vi "SetClosedChannels.vi"(7 "Slot":T1, 8 "Error In":errorcluster, 10 "Channels":bool[](array[boolean]), 11 "Keithley 7001 In":refnum<visa-resource-name>) -> (0 "Error Out":errorcluster, 3 "Keithley 7001 Out":refnum<visa-resource-name>)   [LabVIEW 2012, in "Keithley-7001.lvlib"]
uses:
  Keithley-7001.lvlib
  Controls/Slot.ctl
panel:
  # "33"
  # "34"
  # "35"
  # "1"
  # "2"
  # "3"
  # "4"
  # "5"
  # "6"
  # "7"
  # "8"
  # "9"
  # "10"
  # "11"
  # "12"
  # "13"
  # "14"
  # "15"
  # "16"
  # "17"
  # "18"
  # "19"
  # "20"
  # "21"
  # "22"
  # "23"
  # "24"
  # "25"
  # "26"
  # "27"
  # "28"
  # "29"
  # "30"
  # "31"
  # "32"
  # "36"
  # "37"
  # "38"
  # "39"
  # "40"
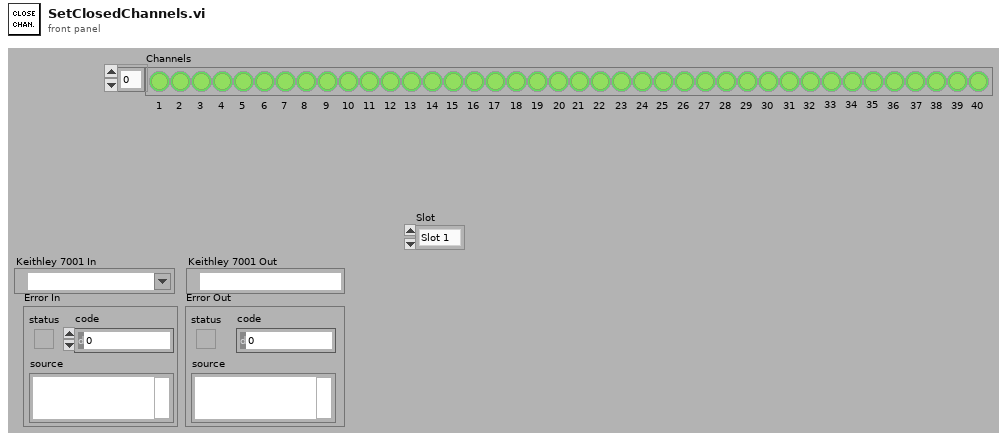
[diagram p1: front panel]
types:
  T1 = typedef "Keithley-7001.lvlib/Slot.ctl" = enum16{"Slot 1", "Slot 2"}
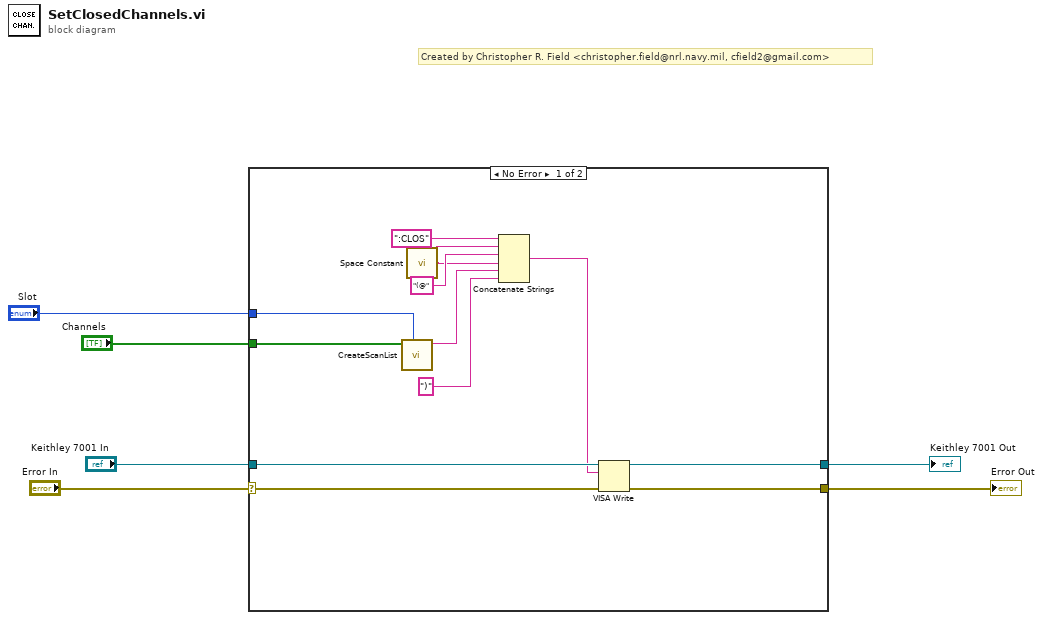
[diagram p0: block diagram]
diagram:
  # "Created by Christopher R. Field <christopher.field@nrl.navy.mil, cfield2@gmail.com>"
  n1 = case shown="No Error" "Error In" {
    selector: "Error In" -> [w8 w19]
    tunnel: "Keithley 7001 In" -> [w18 w20]
    tunnel: [w17 w20] -> w5
    tunnel: [w16 w19] -> w4
    tunnel: "Channels" -> [w13 _]
    tunnel: "Slot" -> [w7 _]
    frame No Error {
      n2 = call "CreateScanList.vi"("Slot"=w7, "Channels"=w13) -> ("Channel List"=w10:string)  [unwired: 9 in]
      n3 = call <vilib>:"Space Constant.vi"() -> ("String"=w11:string)
      n4 = Concatenate Strings(":CLOS", w11, "(@", w11, w10, ")" ("string")) -> (w12:string)
      n5 = VISA Write(VISA resource name=w18, write buffer=w12, error in (no error)=w8) -> (VISA resource name out=w17:refnum<visa-resource-name>, error out=w16:errorcluster)  [unwired: 1 out]
    }
    frame Error {
    }
  }
  "Keithley 7001 Out" <- w5
  "Error Out" <- w4
